vi "Read Selected Shape.vi"(8 "error in (no error)":errorcluster, 11 "Selection in":refnum<class "Selection.lvclass">) -> (0 "error out":errorcluster, 2 "Selected":refnum<data-value>, 3 "Selection out":refnum<class "Selection.lvclass">)   [LabVIEW 2017, in "LV Image Editor Framework.lvlib" / "Selection.lvclass"]
uses:
  <vilib>/LIEF/Forms/Selection/Selection.lvclass
  <vilib>/LIEF/Forms/Shape/Shape.lvclass
  <vilib>/LIEF/Forms/Selection/Selection.lvclass/Selection.ctl
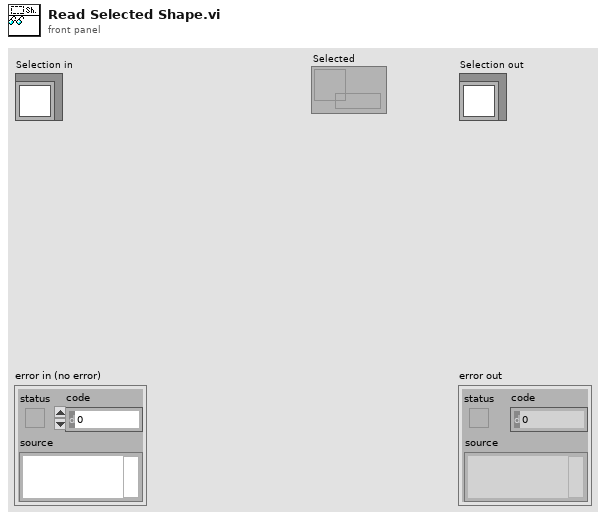
[diagram p1: front panel]
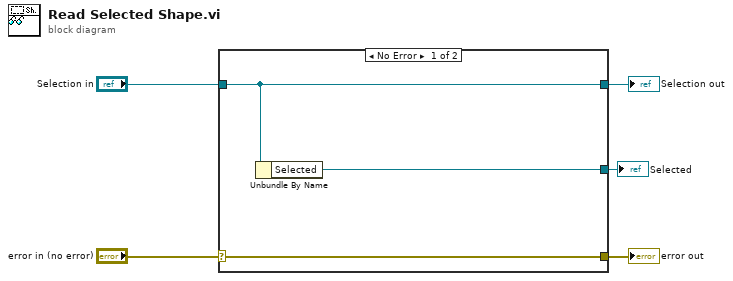
[diagram p0: block diagram]
diagram:
  n1 = case shown="No Error" "error in (no error)" {
    selector: "error in (no error)" -> [w8 w9]
    tunnel: [w8 w9] -> w4
    tunnel: [w7 w10] -> w2
    tunnel: "Selection in" -> [w7 w10]
    tunnel: [w6 _] -> w1
    frame No Error {
      n2 = Unbundle By Name(w7) -> ("Selected"=w6:refnum<data-value>)
    }
    frame Error {
    }
  }
  "error out" <- w4
  "Selection out" <- w2
  "Selected" <- w1
